vi "Configure Analog Gen DC.vi"(7 "Enable Waveform (T: Enable)":bool=TRUE, 8 "error in (no error)":errorcluster, 9 "Amplitude (0 Vp)":dbl, 10 "Channel (0: A)":i32(ring) items=["A", "B"], 11 "VISA resource name":refnum<visa-resource-name>) -> (0 "error out":errorcluster, 3 "VISA resource name out":refnum<visa-resource-name>)   [LabVIEW 2014, in "Stanford Research SR1.lvlib"]
doc: "Configures the attributes for the Analog Generator DC waveform."
uses:
  Stanford Research SR1.lvlib
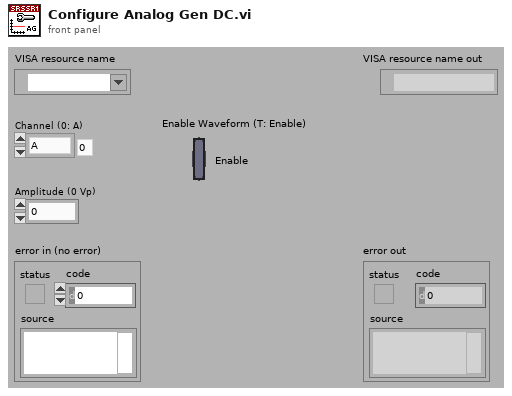
[diagram p1: front panel]
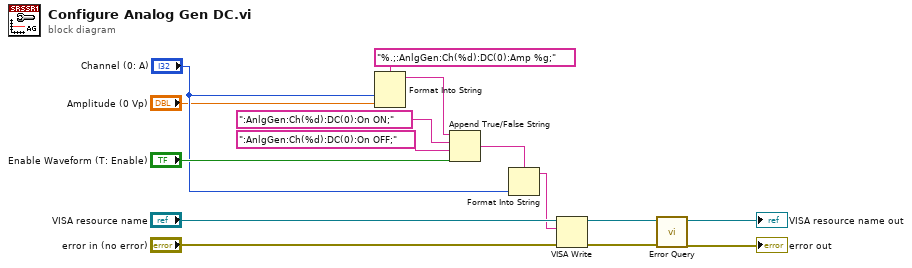
[diagram p0: block diagram]
diagram:
  n1 = Format Into String(format string="%.;:AnlgGen:Ch(%d):DC(0):Amp %g;", "Channel (0: A)", "Amplitude (0 Vp)") -> (resulting string=w14:string)  [unwired: 2 in, 1 out]
  n2 = Append True/False String(1:"Enable Waveform (T: Enable)", 2:":AnlgGen:Ch(%d):DC(0):On OFF;", 3:":AnlgGen:Ch(%d):DC(0):On ON;", 4:w14) -> (0:w4:string)
  n3 = Format Into String(format string=w4, "Channel (0: A)") -> (resulting string=w3:string)  [unwired: 2 in, 1 out]
  n4 = VISA Write(VISA resource name="VISA resource name", write buffer=w3, error in (no error)="error in (no error)") -> (VISA resource name out=w8:refnum<visa-resource-name>, error out=w7:errorcluster)  [unwired: 1 out]
  n5 = call "Error Query.vi"("error in (no error)"=w7, "VISA resource name"=w8) -> ("error out"=→"error out":errorcluster, "VISA resource name out"=→"VISA resource name out":refnum<visa-resource-name>)  [unwired: 6 in, 2 out]
